vi "test median.vi"() -> ()   [LabVIEW 2019]
panel:
  in  "Set Points":dbl[](array[numeric])
  out "output value":dbl
  in  "stop":bool
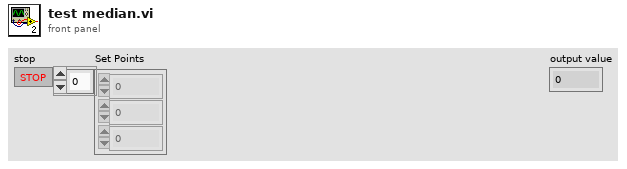
[diagram p1: front panel]
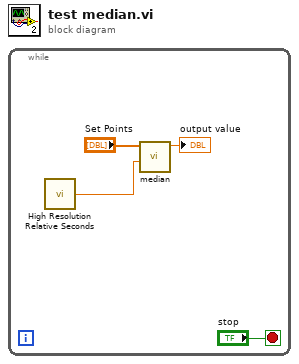
[diagram p0: block diagram]
diagram:
  n1 = while {
    stop <- "stop" stop-if-true
    n2 = call <vilib>:"High Resolution Relative Seconds.vi"() -> ("relative seconds"=w2:dbl)
    n3 = call "median.vi"("Time"=w2, "Set Points"="Set Points") -> ("output value"=→"output value":dbl)  [unwired: 4 in, 1 out]
  }
